vi "Distance Inches to String.vi"(1 "Distance Inches":dbl) -> (0 "Distance String":string)   [LabVIEW 2013]
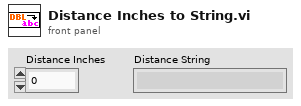
[diagram p1: front panel]
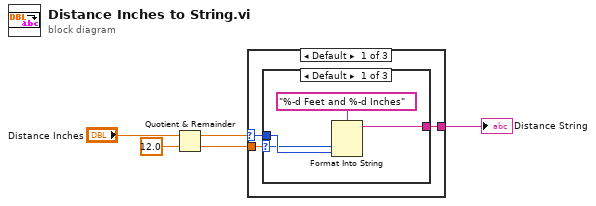
[diagram p0: block diagram]
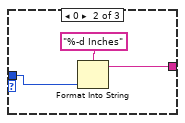
[diagram p2: hidden frame]
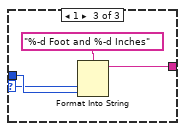
[diagram p3: hidden frame]
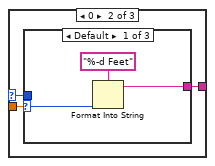
[diagram p4: hidden frame]
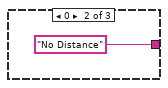
[diagram p5: hidden frame]
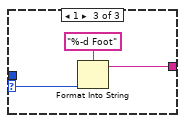
[diagram p6: hidden frame]
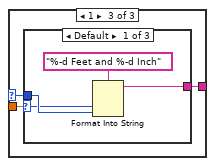
[diagram p7: hidden frame]
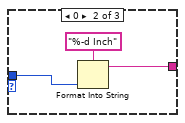
[diagram p8: hidden frame]
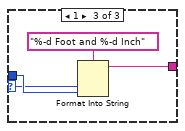
[diagram p9: hidden frame]
diagram:
  n1 = Quotient & Remainder(x="Distance Inches", y=12.0) -> (x-y*floor(x/y)=w3:dbl, floor(x/y)=w2:dbl)
  n2 = case shown="Default" w3 {
    selector: w3 -> [w8 w22 w32]
    tunnel: w2 -> [w7 w21 w31]
    tunnel: [w6 w20 w30] -> w1
    frame Default {
      n3 = case shown="Default" w7 {
        selector: w7 -> [w10 _ w17]
        tunnel: w8 -> [w11 w13 w18]
        tunnel: [w9 w14 w16] -> w6
        frame Default {
          n4 = Format Into String(format string="%-d Feet and %-d Inches", w10, w11) -> (resulting string=w9:string)  [unwired: 2 in, 1 out]
        }
        frame 0 {
          n5 = Format Into String(format string="%-d Inches", w13) -> (resulting string=w14:string)  [unwired: 2 in, 1 out]
        }
        frame 1 {
          n6 = Format Into String(format string="%-d Foot and %-d Inches", w17, w18) -> (resulting string=w16:string)  [unwired: 2 in, 1 out]
        }
      }
    }
    frame 0 {
      n7 = case shown="Default" w21 {
        selector: w21 -> [w24 _ w28]
        tunnel: w22 -> [_ _ _]
        tunnel: [w23 "No Distance" ("format string") w27] -> w20
        frame Default {
          n8 = Format Into String(format string="%-d Feet", w24) -> (resulting string=w23:string)  [unwired: 2 in, 1 out]
        }
        frame 0 {
        }
        frame 1 {
          n9 = Format Into String(format string="%-d Foot", w28) -> (resulting string=w27:string)  [unwired: 2 in, 1 out]
        }
      }
    }
    frame 1 {
      n10 = case shown="Default" w31 {
        selector: w31 -> [w34 _ w41]
        tunnel: w32 -> [w35 w37 w42]
        tunnel: [w33 w38 w40] -> w30
        frame Default {
          n11 = Format Into String(format string="%-d Feet and %-d Inch", w34, w35) -> (resulting string=w33:string)  [unwired: 2 in, 1 out]
        }
        frame 0 {
          n12 = Format Into String(format string="%-d Inch", w37) -> (resulting string=w38:string)  [unwired: 2 in, 1 out]
        }
        frame 1 {
          n13 = Format Into String(format string="%-d Foot and %-d Inch", w41, w42) -> (resulting string=w40:string)  [unwired: 2 in, 1 out]
        }
      }
    }
  }
  "Distance String" <- w1
